vi "Set X-axis.vi"(9 "Times":u32[](array[numeric])) -> (1 "X-label":string, 3 "Multiplier":dbl, 4 "X-Scale Maximum":dbl)   [LabVIEW 2009]
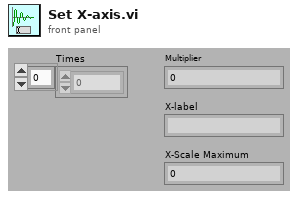
[diagram p1: front panel]
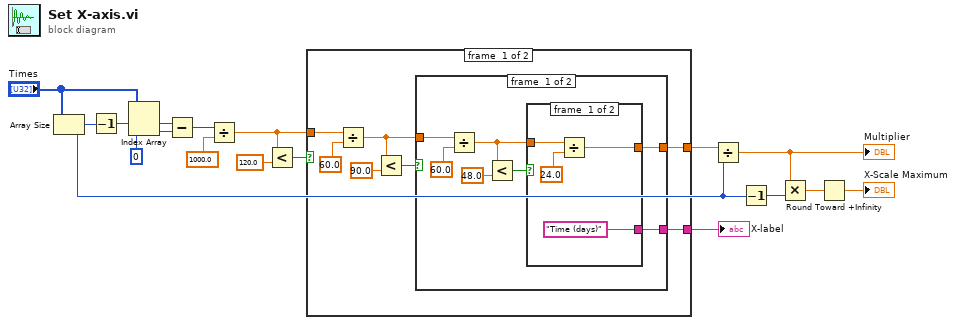
[diagram p0: block diagram]
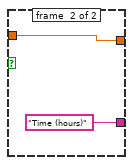
[diagram p2: hidden frame]
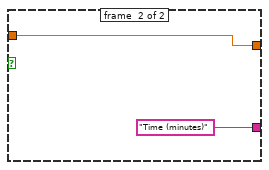
[diagram p3: hidden frame]
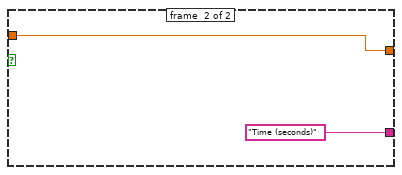
[diagram p4: hidden frame]
diagram:
  n1 = Array Size(array="Times") -> (size(s)=w5:i32)
  n2 = Decrement(x=w5) -> (x-1=w6:i32)
  n3 = Index Array(array="Times", index #1=w6, index #2=0 ("index")) -> (element #1=w9:u32, element #2=w10:u32)
  n4 = Subtract(x=w9, y=w10) -> (x-y=w14:u32)
  n5 = Divide(x=w14, y=1000.0 ("index")) -> (x/y=w15:dbl)
  n6 = Less?(x=w15, y=120.0) -> (x < y?=w13:bool)
  n7 = case shown="False" w13 {
    tunnel: w15 -> [w22 w41]
    tunnel: [w19 w41] -> w16
    tunnel: [w18 "Time (seconds)"] -> w17
    frame #0 {
      n8 = Divide(x=w22, y=60.0 ("index")) -> (x/y=w20:dbl)
      n9 = Less?(x=w20, y=90.0) -> (x < y?=w21:bool)
      n10 = case shown="False" w21 {
        tunnel: w20 -> [w29 w39]
        tunnel: [w26 w39] -> w19
        tunnel: [w25 "Time (minutes)"] -> w18
        frame #0 {
          n11 = Divide(x=w29, y=60.0 ("index")) -> (x/y=w27:dbl)
          n12 = Less?(x=w27, y=48.0) -> (x < y?=w28:bool)
          n13 = case shown="False" w28 {
            tunnel: w27 -> [w34 w36]
            tunnel: [w32 w36] -> w26
            tunnel: ["Time (days)" "Time (hours)"] -> w25
            frame #0 {
              n14 = Divide(x=w34, y=24.0 ("index")) -> (x/y=w32:dbl)
            }
            frame #1 {
            }
          }
        }
        frame #1 {
        }
      }
    }
    frame #1 {
    }
  }
  "X-label" <- w17
  n15 = Divide(x=w16, y=w5) -> (x/y=w3:dbl)
  "Multiplier" <- w3
  n16 = Decrement(x=w5) -> (x-1=w4:i32)
  n17 = Multiply(x=w3, y=w4) -> (x*y=w2:dbl)
  n18 = Round Toward +Infinity(x=w2) -> (ceil(x): smallest int >= x=→"X-Scale Maximum":dbl)
